vi "keyence ethernet ip tester.vi"() -> ()   [LabVIEW 2018]
panel:
  in  "Network Path":string="172.15.51.158"
  out "error out":errorcluster
  in  "update preset":bool
  out "zero offset":dbl
  in  "Preset Command":dbl
  out "PV":dbl format="%#.3g"
  in  "Instance ID in  (LVDT Amplifier Index [1..n])":u32=1
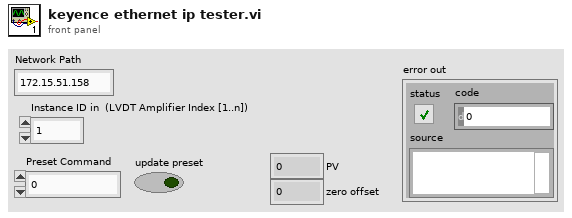
[diagram p1: front panel]
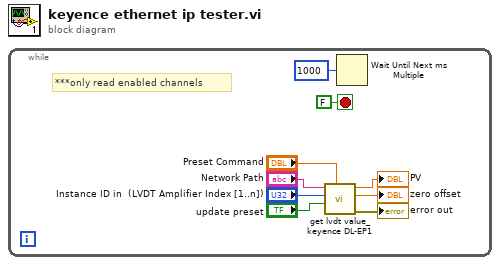
[diagram p0: block diagram]
diagram:
  n1 = while {
    stop <- FALSE stop-if-true
    # "***only read enabled channels"
    n2 = call "get lvdt value_keyence DL-EP1.vi"("Preset Command"="Preset Command", "update preset"="update preset", "Instance ID in  (LVDT Amplifier Index [1..n])"="Instance ID in  (LVDT Amplifier Index [1..n])", "Network Path"="Network Path") -> ("error out"=→"error out":errorcluster, "Zero-Offset"=→"zero offset":dbl, "PV"=→"PV":dbl)  [unwired: 5 in]
    n3 = Wait Until Next ms Multiple(millisecond multiple=u32 1000) -> ()  [unwired: 1 out]
  }
